vi "Write Data.vi"(0 "comm interface in":refnum<class "RoboRIO SPI.lvclass">, 5 "data":u8[](array[numeric]), 11 "error in":errorcluster) -> (4 "comm interface out":refnum<class "RoboRIO SPI.lvclass">, 15 "error out":errorcluster)   [LabVIEW 2018, in "RoboRIO SPI.lvclass"]
uses:
  RoboRIO SPI.lvclass
  RoboRIO SPI.lvclass/RoboRIO SPI.ctl
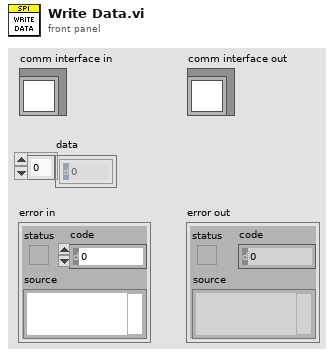
[diagram p1: front panel]
types:
  T1 = typedef "WPI_SPIDevRef.ctl" = cluster{"DevStatus":errorcluster, "Handle":i32, "SPI Bus":T2}
  T2 = typedef "spi_bus.ctl" = enum16{"SPI On-Board, CS0", "SPI On-Board, CS1", "SPI On-Board, CS2", "SPI On-Board, CS3", "SPI MXP", "Invalid"}
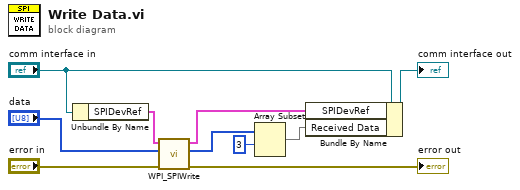
[diagram p0: block diagram]
diagram:
  n1 = Unbundle By Name("comm interface in") -> ("SPIDevRef"=w7:T1)
  n2 = call <vilib>:"WPI_SPIWrite.vi"("error in (no error)"="error in", "Data To Send"="data", "SPIDevRef"=w7) -> ("error out"=→"error out":errorcluster, "Received Data"=w3:u8[], "SPIDevRef"=w8:T1)  [unwired: 6 in]
  n3 = Array Subset(array=w3, index=3) -> (w2:u8[])  [unwired: 1 in]
  n4 = Bundle By Name(cluster="comm interface in", "SPIDevRef"=w8, "Received Data"=w2) -> (→"comm interface out":refnum<class "RoboRIO SPI.lvclass">)
